vi "File Action V1.vi"(0 "Action":string, 2 "Mode":u16(ring) items=["Read", "Write"], 7 "Image Acquisition Parameters Array":T1[](array[typedef]) {"Z Steps Size (um)" min=0.0; "Number of Z Steps" min=1; "Frames Accumulations" min=1; "Frames Per Capture" min=1; "Line Accumulations" min=1; "Image Format" items=["64 x 64"=64, "128 x 128"=128, "256 x 256"=256, "512 x 512"=512, "1024 x 1024"=1024, "2048 x 2048"=2048]}, 11 "File Path IN":path, 13 "Number of Channels":i32) -> (4 "File Path OUT":path, 8 "File REFs":refnum<file>[](array[refnum]), 15 "Files Open":bool)   [LabVIEW 2016]
uses:
  Type Defs/Image Acquisition Parameters.ctl
  Write TIFF/ImageJ TIF Type Defs/TIF Write Image Information.ctl
panel:
  # "Copyright (C) 2020 Edward S Allgeyer\n\nRedistribution and use in source and binary forms, with or without\nmodification, are permitted provided that the following conditions\nare met:\n\n1. Redistributions of source code must retain the above copyright\n   notice, this list of conditions and the following disclaimer.\n\n2. Redistributions in binary form must reproduce the above copyright\n   notice, this list of conditions and the following disclaimer in\n   the documentation and/or other materials provided with the\n   distribution.\n\n3. Neither the name of the copyright holder nor the names of its\n   contributors may be used to endorse or promote products derived\n   from this software without specific prior written permission.\n\nTHIS SOFTWARE IS PROVIDED BY THE COPYRIGHT HOLDERS AND CONTRIBUTORS\n\"AS IS\" AND ANY EXPRESS OR IMPLIED WARRANTIES, INCLUDING, BUT NOT\nLIMITED TO, THE IMPLIED WARRANTIES OF MERCHANTABILITY AND FITNESS\nFOR A PARTICULAR PURPOSE ARE DISCLAIMED. IN NO EVENT SHALL THE\nCOPYRIGHT HOLDER OR CONTRIBUTORS BE LIABLE FOR ANY DIRECT, INDIRECT,\nINCIDENTAL, SPECIAL, EXEMPLARY, OR CONSEQUENTIAL DAMAGES (INCLUDING,\nBUT NOT LIMITED TO, PROCUREMENT OF SUBSTITUTE GOODS OR SERVICES;\nLOSS OF USE, DATA, OR PROFITS; OR BUSINESS INTERRUPTION) HOWEVER\nCAUSED AND ON ANY THEORY OF LIABILITY, WHETHER IN CONTRACT, STRICT\nLIABILITY, OR TORT (INCLUDING NEGLIGENCE OR OTHERWISE) ARISING IN\nANY WAY OUT OF THE USE OF THIS SOFTWARE, EVEN IF ADVISED OF THE\nPOSSIBILITY OF SUCH DAMAGE."
  # "XY"
  # "Z"
  # "Length"
  # "Height"
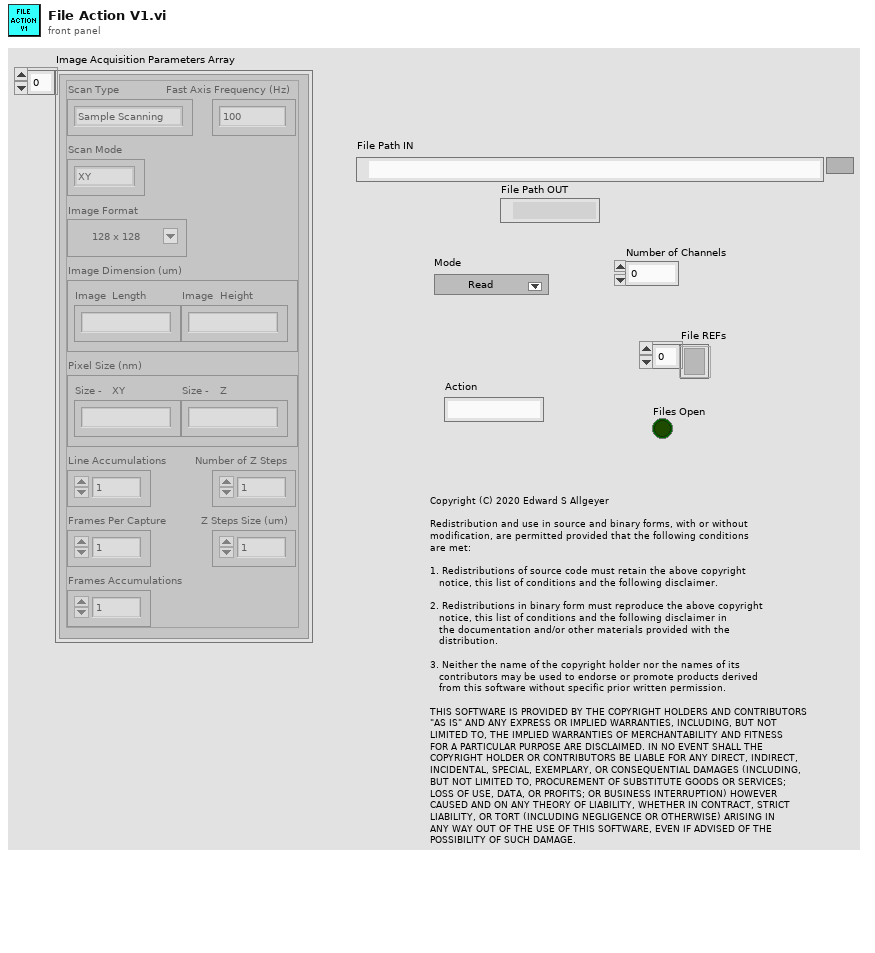
[diagram p1: front panel]
types:
  T1 = typedef "Image Acquisition Parameters.ctl" = cluster{"Scan Type":enum16{"Sample Scanning", "Beam Scanning"}, "Scan Mode":enum16{"XY", "XZ", "YZ", "XYZ"}, "Fast Axis Frequency (Hz)":dbl, "Image Format":u16, "Line Accumulations":u16, "Frames Per Capture":u16, "Frames Accumulations":u16, "Image Dimension (um)":dbl[], "Number of Z Steps":u8, "Z Steps Size (um)":dbl, "Pixel Size (nm)":dbl[]}
  T2 = cluster{"Z Length (um)":sgl, "Y Length (um)":sgl, "X Length (um)":sgl, "t (s)":sgl}
  T3 = typedef "TIF Write Image Information.ctl" = cluster{"Image Width (Pixels)":u32, "Image Height (Pixels)":u32, "Pixel Width (µm)":dbl, "Pixel Height (µm)":dbl, "Bits Per Sample (e.g. 16)":u32, "No. of Frames":u32, "No. of Slices":u32, "Time Step (sec)":dbl, "Z Step (µm)":dbl}
  T4 = cluster{"Number of Z Steps":u8, "Image Format":u16, "Image Format":u16, "Frames Per Capture":u16}
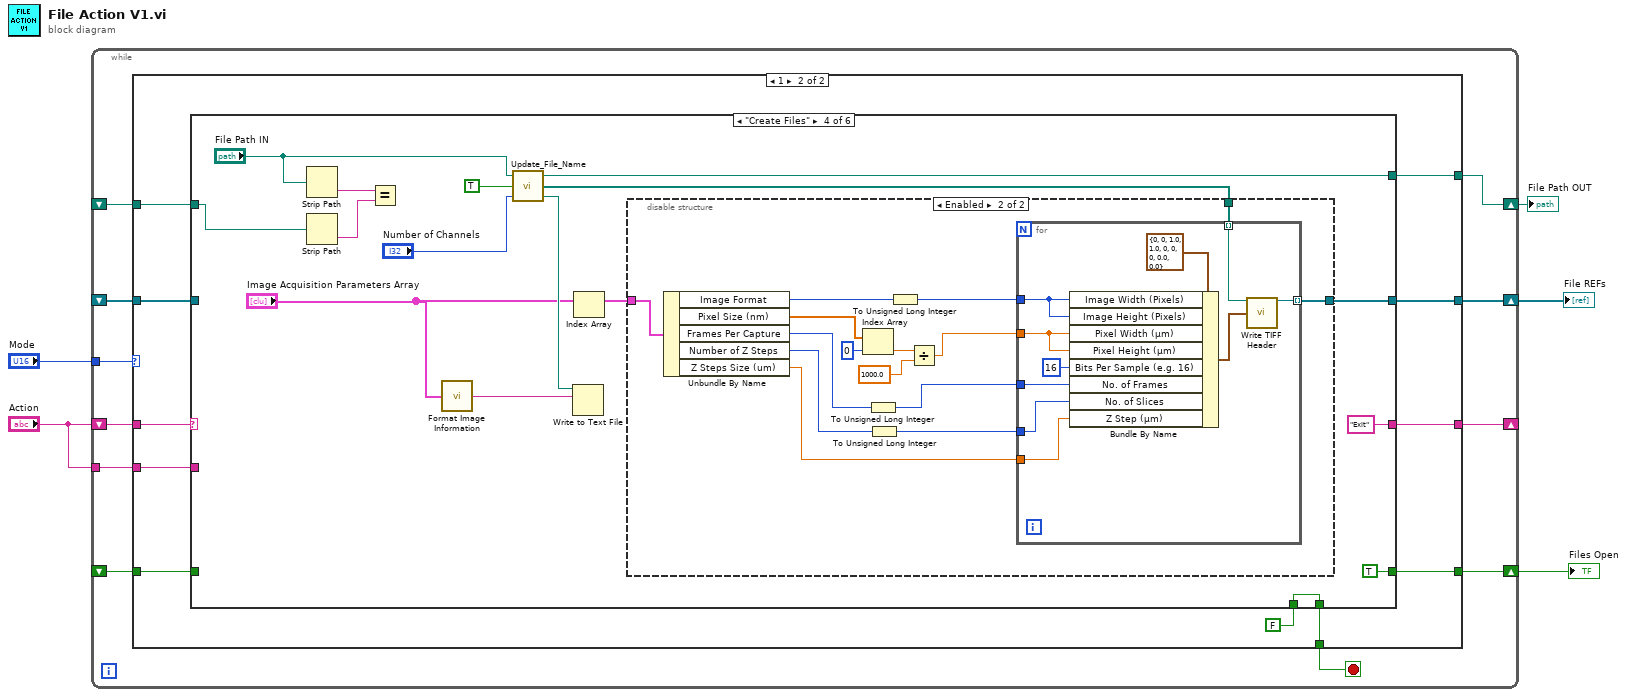
[diagram p0: block diagram]
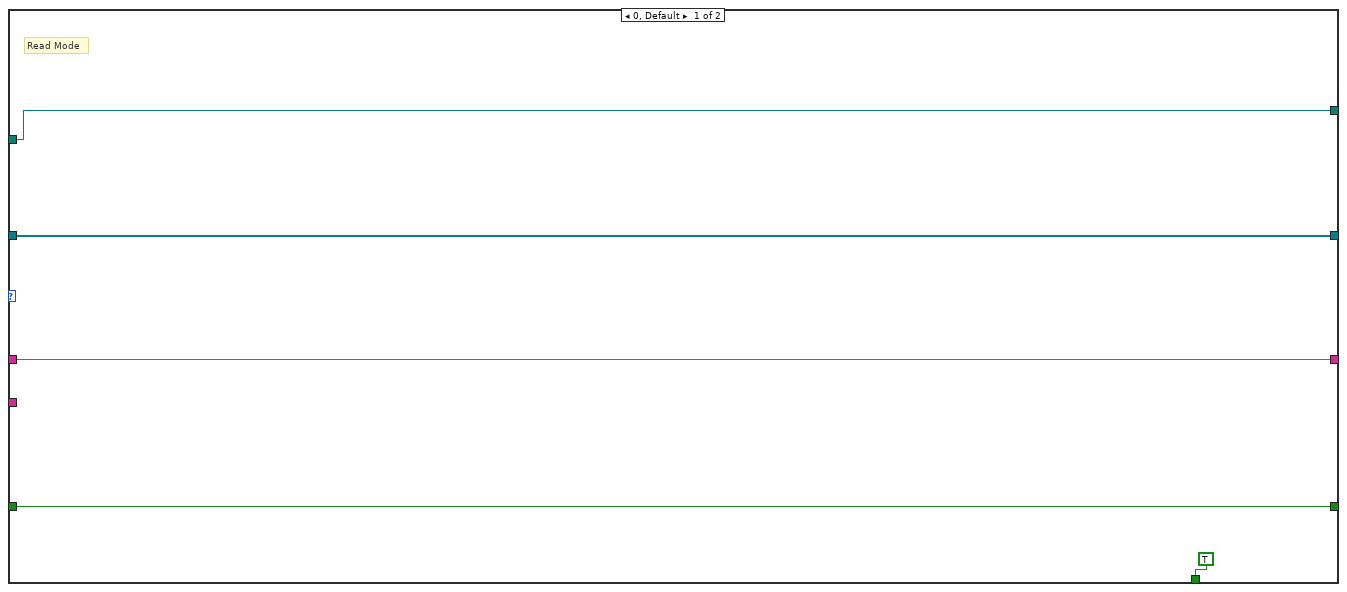
[diagram p2: hidden frame]
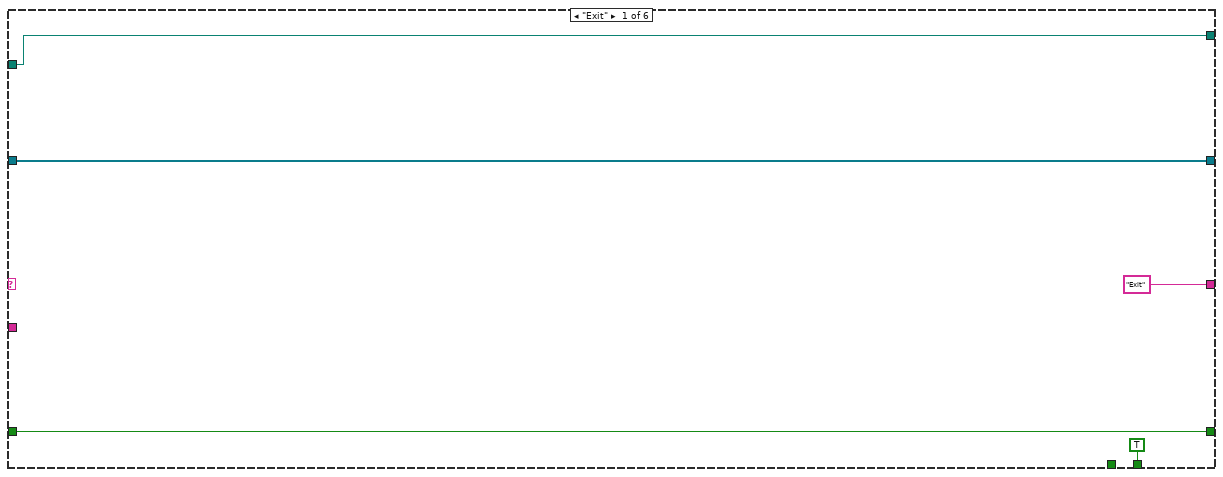
[diagram p3: hidden frame]
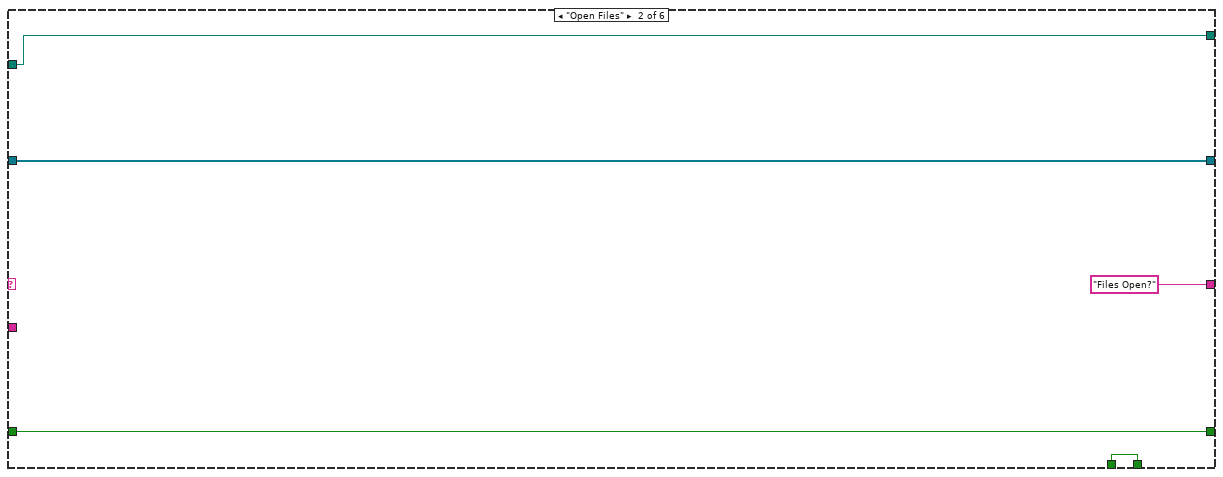
[diagram p4: hidden frame]
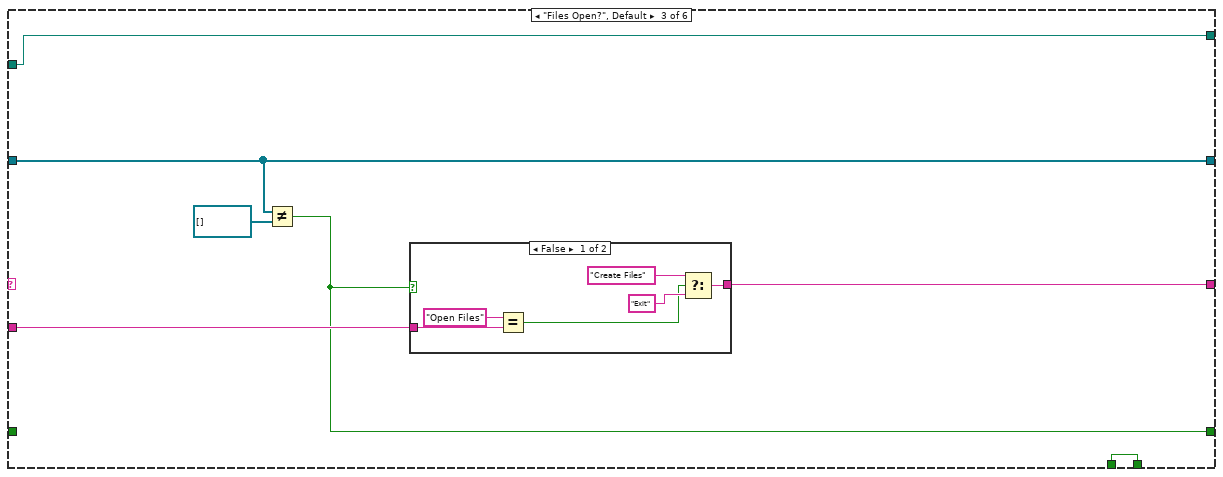
[diagram p5: hidden frame]
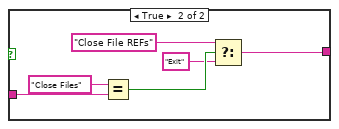
[diagram p6: hidden frame]
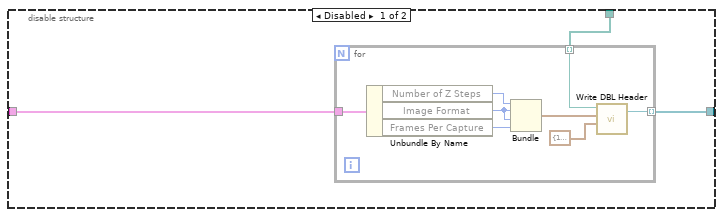
[diagram p7: hidden frame]
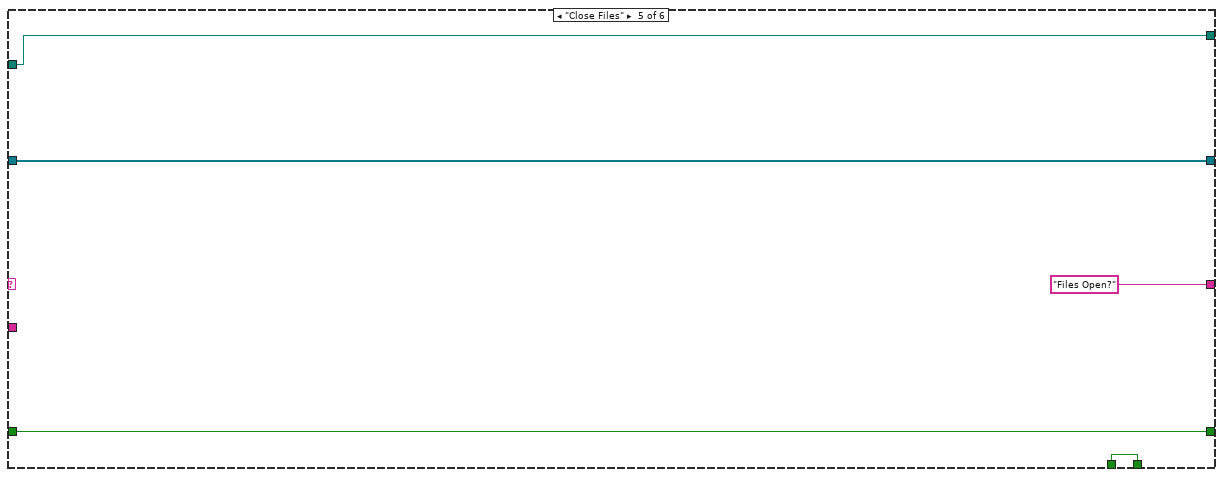
[diagram p8: hidden frame]
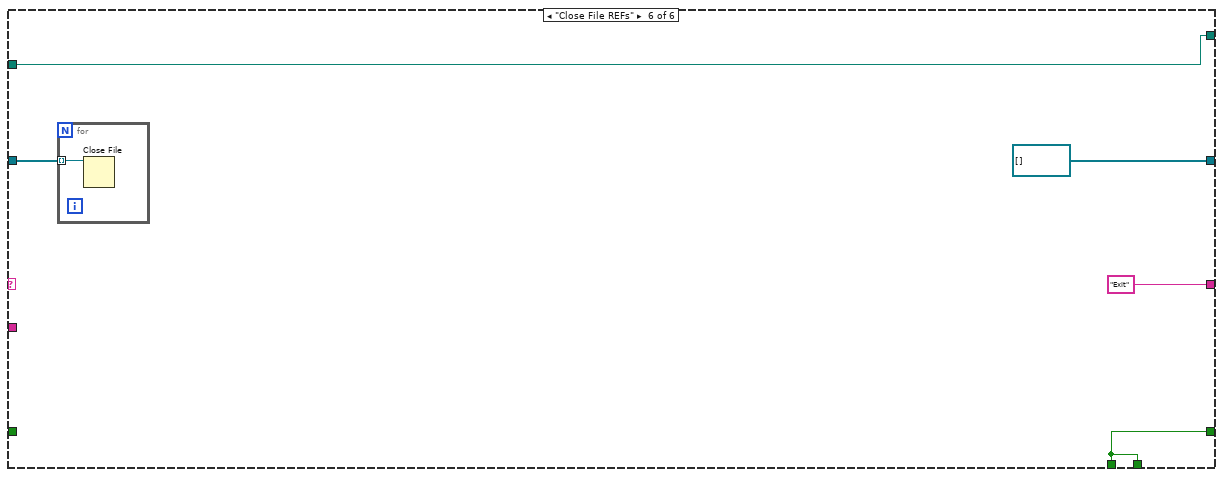
[diagram p9: hidden frame]
diagram:
  n1 = while {
    tunnel: "Mode" -> [w16]
    shift-right: [w15] -> w4
    shift-left: _ -> [w14]
    shift-right: [w12] -> _
    shift-left: "Action" -> [w13]
    tunnel: "Action" -> [w10]
    shift-right: [w9] -> w2
    shift-left: _ -> [w8]
    shift-right: [w7] -> w1
    shift-left: _ -> [w6]
    stop <- w11 stop-if-true
    n2 = case shown="1" w16 {
      tunnel: [w21 w32] -> w15
      tunnel: w14 -> [w21 w30]
      tunnel: w13 -> [w20 w31]
      tunnel: [w20 w29] -> w12
      tunnel: [TRUE w26] -> w11
      tunnel: w10 -> [_ w28]
      tunnel: [w18 w25] -> w9
      tunnel: w8 -> [w18 w24]
      tunnel: [w17 w23] -> w7
      tunnel: w6 -> [w17 w22]
      frame 0, Default {
        # "Read Mode"
      }
      frame 1 {
        n3 = case shown="\"Create Files\"" w31 {
          tunnel: [w35 w42 w48 w71 w118 refnum<file>[] []] -> w32
          tunnel: w30 -> [w35 w42 w48 _ w118 w123]
          tunnel: ["Exit" "Files Open?" w47 "Exit" "Files Open?" "Exit"] -> w29
          tunnel: w28 -> [_ _ w46 _ _ _]
          tunnel: FALSE -> [_ w40 w45 w77 w116 w120]
          tunnel: [TRUE w40 w45 w77 w116 w120] -> w26
          tunnel: [w34 w39 w44 TRUE w115 w120] -> w25
          tunnel: w24 -> [w34 w39 _ _ w115 _]
          tunnel: [w33 w38 w43 w70 w114 w119] -> w23
          tunnel: w22 -> [w33 w38 w43 w67 w114 w119]
          frame "Exit" {
          }
          frame "Open Files" {
          }
          frame "Files Open?", Default {
            n4 = Not Equal?(x=w48, y=refnum<file>[] []) -> (x != y?=w44:bool)
            n5 = case shown="False" w44 {
              tunnel: [w51 w58] -> w47
              tunnel: w46 -> [w55 w60]
              frame False {
                n6 = Equal?(x="Open Files", y=w55) -> (x = y?=w50:bool)
                n7 = Select(t="Create Files", s=w50, f="Exit") -> (s? t:f=w51:string)
              }
              frame True {
                n8 = Equal?(x="Close Files", y=w60) -> (x = y?=w59:bool)
                n9 = Select(t="Close File REFs", s=w59, f="Exit") -> (s? t:f=w58:string)
              }
            }
          }
          frame "Create Files" {
            n10 = Strip Path(path="File Path IN") -> (name=w65:string)  [unwired: 1 out]
            n11 = Strip Path(path=w67) -> (name=w64:string)  [unwired: 1 out]
            n12 = Equal?(x=w65, y=w64) -> ()  [unwired: 1 out]
            n13 = call "Format Image Information.vi"("Image Acquisition Parameters Array"="Image Acquisition Parameters Array") -> ("Result"=w74:string)  [unwired: 14 in]
            n14 = call "Update_File_Name.vi"("Number of Channels"="Number of Channels", "New File"=TRUE, "File Path IN"="File Path IN") -> ("Text Image Data Path"=w73:path, "File References"=w72:path[], "File Path OUT"=w70:path)
            n15 = Write to Text File(file (use dialog)=w73, text=w74) -> ()  [unwired: 2 in, 3 out]
            n16 = Index Array(array="Image Acquisition Parameters Array") -> (element=w68:T1)  [unwired: 1 in]
            n17 = disable-structure shown="Enabled" {
              disable-tunnel: w72 -> [w80 w103]
              disable-tunnel: [w79 w102] -> w71
              disable-tunnel: w68 -> [w78 w101]
              frame Disabled {
                n18 = for {
                  tunnel: w78 -> [w85]
                  tunnel: w80 -> [w82] mode=indexing
                  tunnel: [w81] -> w79 mode=indexing
                  n19 = Unbundle By Name(w85) -> ("Number of Z Steps"=w83:u8, "Image Format"=w87:u16, "Frames Per Capture"=w84:u16)
                  n20 = Bundle("Number of Z Steps"=w83, "Image Format"=w87, "Image Format"=w87, "Frames Per Capture"=w84) -> (w86:T4)  [unwired: 1 in]
                  n21 = call "Write DBL Header.vi"("Physical Lengths (um)"=T2 {"Z Length (um)"=1.0, "Y Length (um)"=1.0, "X Length (um)"=1.0, "t (s)"=1.0}, "Pixel Lengths"=w86, "File Path IN"=w82) -> ("File Ref OUT"=w81:refnum<file>)  [unwired: 1 in, 1 out]
                }
              }
              frame Enabled {
                n22 = Unbundle By Name(w101) -> ("Image Format"=w100:u16, "Pixel Size (nm)"=w98:dbl[], "Frames Per Capture"=w93:u16, "Number of Z Steps"=w91:u8, "Z Steps Size (um)"=w89:dbl)
                n23 = Index Array(array=w98, index=0) -> (element=w96:dbl)
                n24 = To Unsigned Long Integer(number=w93) -> (unsigned 32bit integer=w92:u32)
                n25 = To Unsigned Long Integer(number=w91) -> (unsigned 32bit integer=w90:u32)
                n26 = To Unsigned Long Integer(number=w100) -> (unsigned 32bit integer=w99:u32)
                n27 = Divide(x=w96, y=1000.0) -> (x/y=w94:dbl)
                n28 = for {
                  tunnel: w103 -> [w113] mode=indexing
                  tunnel: [w112] -> w102 mode=indexing
                  tunnel: w99 -> [w109]
                  tunnel: w94 -> [w108]
                  tunnel: w92 -> [w106]
                  tunnel: w90 -> [w105]
                  tunnel: w89 -> [w104]
                  n29 = Bundle By Name(cluster=T3 {"Image Width (Pixels)"=0, "Image Height (Pixels)"=0, "Pixel Width (µm)"=1.0, "Pixel Height (µm)"=1.0, "Bits Per Sample (e.g. 16)"=0, "No. of Frames"=0, "No. of Slices"=0, "Time Step (sec)"=0.0, "Z Step (µm)"=0.0} ("Image Info"), "Image Width (Pixels)"=w109, "Image Height (Pixels)"=w109, "Pixel Width (µm)"=w108, "Pixel Height (µm)"=w108, "Bits Per Sample (e.g. 16)"=u32 16, "No. of Frames"=w106, "No. of Slices"=w105, "Z Step (µm)"=w104) -> (w110:T3)
                  n30 = call "Write TIFF Header.vi"("File Path"=w113, "Image Info"=w110) -> ("File Ref"=w112:refnum<file>)  [unwired: 11 in, 2 out]
                }
              }
            }
          }
          frame "Close Files" {
          }
          frame "Close File REFs" {
            n31 = for {
              tunnel: w123 -> [w124] mode=indexing
              n32 = Close File(refnum=w124) -> ()  [unwired: 1 in, 2 out]
            }
          }
        }
      }
    }
  }
  "File REFs" <- w4
  "Files Open" <- w2
  "File Path OUT" <- w1
